vi "Add Item to Tree.vi"(8 "error in (no error)":errorcluster, 10 "Dynamic Dispatch VI Type in":refnum<class "Dynamic Dispatch VI Type.lvclass">, 11 "Tree Ref in":refnum<vi>) -> (0 "error out":errorcluster, 1 "Added Tag":string, 2 "Dynamic Dispatch VI Type out":refnum<class "Dynamic Dispatch VI Type.lvclass">, 3 "Tree Ref out":refnum<vi>)   [LabVIEW 2020, in "Peek Window.lvlib" / "Dynamic Dispatch VI Type.lvclass"]
uses:
  Dynamic Dispatch VI Type.lvclass
  D:/Code/VI-Peek/source/Peek Window/VI Types/Standard VI Type/Standard VI Type.lvclass
  Symbols Enum.ctl
  Standard VI Type/Standard VI Type.lvclass/Standard VI Type.ctl
  Standard VI Type/Read Selectable.vi
  Standard VI Type/Read Full Qualified Name.vi
  Dynamic Dispatch VI Type.lvclass/Dynamic Dispatch VI Type.ctl
  Peek Window.lvlib
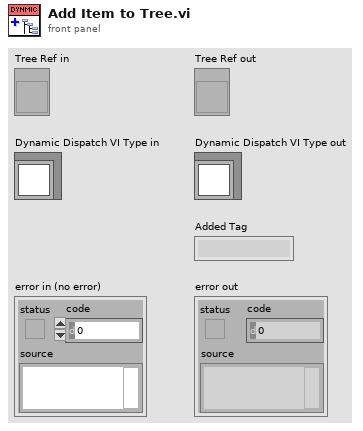
[diagram p1: front panel]
types:
  T1 = typedef "Peek Window.lvlib/Symbols Enum.ctl" = enum16{"<Blank>", "Below Here Glyph", "VI", "Dynamic Dispatch VI", "Malleable VI", "Polymorphic VI", "Missing VI", "Express VI"}
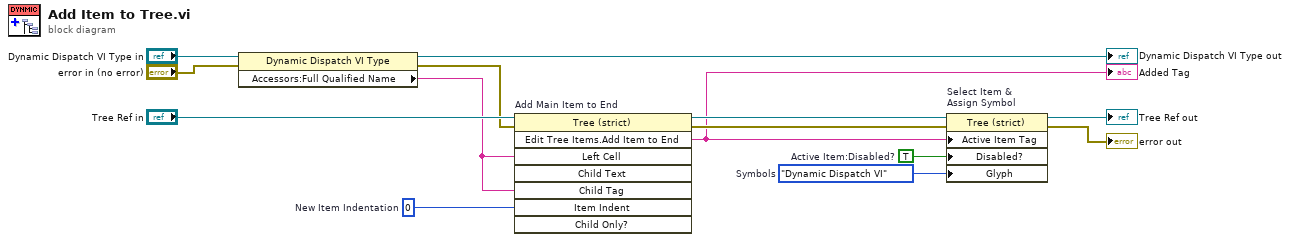
[diagram p0: block diagram]
diagram:
  w1 = TRUE  # Active Item:Disabled?
  w11 = Symbols_Enum."Dynamic Dispatch VI"  # Symbols
  w14 = 0  # New Item Indentation
  n1 = property class="Dynamic Dispatch VI Type"(reference="Dynamic Dispatch VI Type in", error in="error in (no error)") -> (reference out=→"Dynamic Dispatch VI Type out":refnum<class "Dynamic Dispatch VI Type.lvclass">, error out=w8:errorcluster, "Accessors:Full Qualified Name"=w4:string)
  n2 = invoke on="Add Main Item to End" class="Tree (strict)" method="Edit Tree Items.Add Item to End"(reference="Tree Ref in", error in=w8, "Left Cell"=w4, "Child Tag"=w4, "Item Indent"=w14) -> (reference out=w13:refnum<vi>, error out=w12:errorcluster, "Edit Tree Items:Add Item to End"=w7:string)  [unwired: 3 in, 5 out]
  "Added Tag" <- w7
  n3 = property on="Select Item &\nAssign Symbol" class="Tree (strict)"(reference=w13, error in=w12, "Active Item Tag"=w7, "Disabled?"=w1, "Glyph"=w11) -> (reference out=→"Tree Ref out":refnum<vi>, error out=→"error out":errorcluster)
